vi "Update.vi"(8 "error in (no error)":errorcluster, 10 "Message in":refnum<class "UpdateMessage.lvclass">, 11 "Template in":refnum<class "Template.lvclass">) -> (0 "error out":errorcluster, 3 "Template out":refnum<class "Template.lvclass">)   [LabVIEW 2012, in "Template.lvclass"]
doc: "The update method processes the command 'update'. \n\nThe command 'update' is used for receiving new values to be set to the private data of the class. This could be seen as a public set method for setting new parameters to the private class data."
uses:
  Template.lvclass
  <vilib>/Distrio/Murmex/UpdateMessage/UpdateMessage.lvclass
  Template.lvclass/Template.ctl
  <vilib>/Distrio/Murmex/Murmex/Murmex.lvclass
panel:
  # "This method is called when the UPDATE\ntrigger is sent. \n\nOverride this method when your component needs to\nrespond to this trigger. \n\nCall parent for proper implementation"
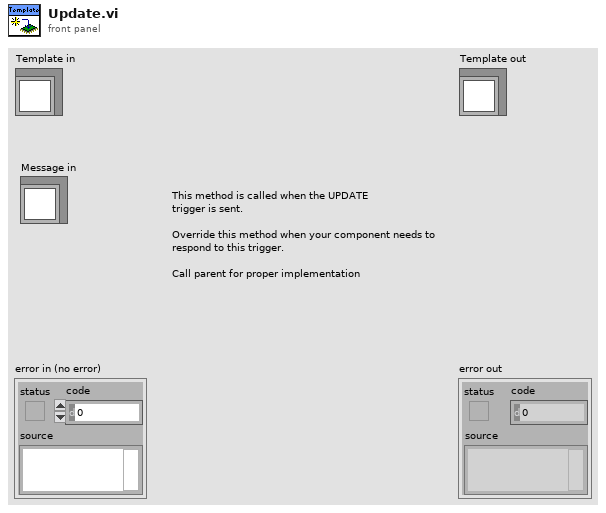
[diagram p1: front panel]
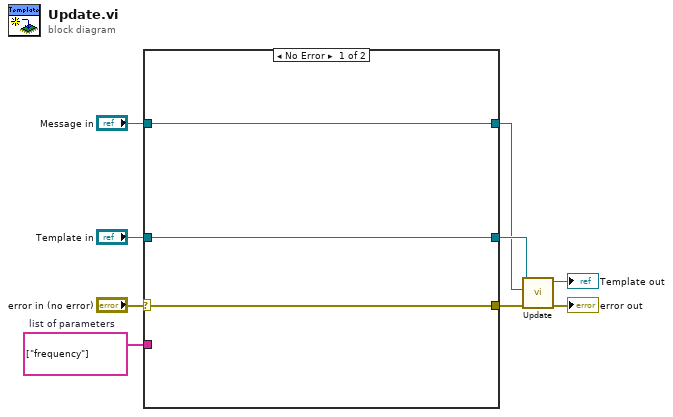
[diagram p0: block diagram]
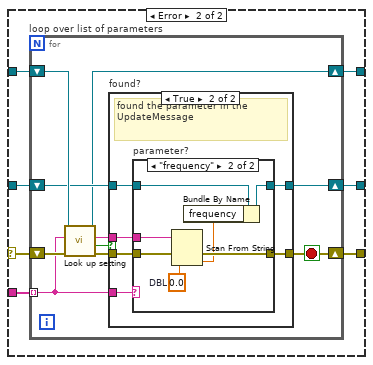
[diagram p2: hidden frame]
diagram:
  w9 = string[] ["frequency"]  # list of parameters
  n1 = case shown="No Error" "error in (no error)" {
    selector: "error in (no error)" -> [w12 w18]
    tunnel: [w12 w17] -> w6
    tunnel: [w11 w14] -> w5
    tunnel: "Message in" -> [w10 w19]
    tunnel: w9 -> [_ w16]
    tunnel: "Template in" -> [w11 w15]
    tunnel: [w10 w13] -> w1
    frame No Error {
    }
    frame Error {
      n2 = for "loop over list of parameters" {
        shift-right: [w23] -> w17
        shift-left: w18 -> [w28]
        tunnel: w16 -> [w24] mode=indexing
        shift-right: [w21] -> w14
        shift-left: w15 -> [w22]
        shift-right: [w20] -> w13
        shift-left: w19 -> [w29]
        stop <- w23 stop-if-true
        n3 = call <vilib>:"Look up setting.vi"("error in (no error)"=w28, "tag name"=w24, "UpdateMessage in"=w29) -> ("error out"=w25:errorcluster, "found?"=w27:bool, "value"=w26:string, "UpdateMessage out"=w20:refnum<class "UpdateMessage.lvclass">)  [unwired: 5 in]
        n4 = case "found?" shown="True" w27 {
          tunnel: w26 -> [_ w37]
          tunnel: w25 -> [w31 w36]
          tunnel: w24 -> [_ w35]
          tunnel: [w31 w34] -> w23
          tunnel: w22 -> [w30 w33]
          tunnel: [w30 w32] -> w21
          frame False {
          }
          frame True {
            # "found the parameter in the UpdateMessage"
            n5 = case "parameter?" shown="\"frequency\"" w35 {
              tunnel: w37 -> [_ w46]
              tunnel: w36 -> [w39 w45]
              tunnel: [w39 w43] -> w34
              tunnel: w33 -> [w38 w42]
              tunnel: [w38 w41] -> w32
              frame Default {
              }
              frame "frequency" {
                w44 = 0.0  # DBL
                n6 = Scan From String(input string=w46, error in=w45, default 1=w44) -> (error out=w43:errorcluster, output 1=w40:dbl)  [unwired: 2 in, 2 out]
                n7 = Bundle By Name(cluster=w42, "frequency"=w40) -> (w41:refnum<class "Template.lvclass">)
              }
            }
          }
        }
      }
    }
  }
  n8 = call-parent "Update.vi"("error in (no error)"=w6, "Message in"=w1, "Murmex in"=w5) -> ("error out"=→"error out":errorcluster, "Murmex out"=→"Template out":refnum<class "Template.lvclass">)  [unwired: 7 in]
